vi "Lab Panel V2.1.vi"() -> ()   [LabVIEW 2013]
uses:
  <vilib>/Platform/TimedLoop/XDataNode/timing_clust.ctl
  <vilib>/Platform/TimedLoop/XDataNode/nitl_modes.ctl
  <vilib>/Platform/TimedLoop/XDataNode/wakeup.ctl
  <vilib>/platform/TimedLoop/XDataNode/XDataNode.xnode
  <vilib>/Platform/TimedLoop/XDataNode/XDNodeRunTimeDep.lvlib
panel:
  in  "Tab Control 2":enum32{"Page 1", "Page 2", "ADMIN"}(tab)
  in  "LA05-2 Name":string
  in  "LA05-1 Name":string
  in  "LA01-1 Testers Name 2":string
  in  "LA01-1 Testers Name":string
  in  "LA01-1 Testers Name 6":string
  in  "LA01-1 Testers Name 5":string
  in  "LA01-1 Testers Name 4":string
  in  "LA01-1 Testers Name 3":string
  in  "LA01-2 Name":string
  in  "LA01-1 Name":string
  out "LA01-1 (V) 10":dbl
  out "LA01-1 (V) 9":dbl
  out "LA01-1 (V) 8":dbl
  out "LA01-1 (V) 7":dbl
  out "LA01-1 (V) 6":dbl
  out "LA01-1 (V) 5":dbl
  out "LA01-1 (V) 4":dbl
  out "LA01-1 (V) 3":dbl
  out "LA01-2 (V)":dbl
  out "LA01-1 (V)":dbl
  in  "Tab Control":T1(tab)
  out "Waveform Graph":dynamicdata(graph)
  out "Waveform Graph 2":dynamicdata(graph)
  out "volt1 4":dbl format="%.2g"
  out "volt1 3":dbl format="%.2g"
  out "volt1 2":dbl format="%.2g"
  out "volt1":dbl format="%.2g"
  out "Waveform Graph 3":dynamicdata(graph)
  out "error out":errorcluster
  in  "Stop Button":bool
  out "AI loop time":dbl format="%.6g"
  out "loops":dbl
  out "saving data":bool
  in  "loop  delay(mS)":dbl
  out "Filename Out":path
  out "on loops":dbl
  in  "on time":dbl=1.0 min=1.0 max=10.0 step=0.5 format="%.1g"
  out "off loops":dbl
  in  "off time":dbl=2.0 min=2.0 max=10.0 step=0.5 format="%.1g"
  out "jig":bool
  out "jig cycle":dbl
  in  "run test":bool
  in  "calibrate":bool
  in  "LA01 TEMP":dbl[](array[numeric])
  in  "LA02 TEMP":dbl[](array[numeric])
  in  "LA03 TEMP":dbl[](array[numeric])
  in  "LA04 TEMP":dbl[](array[numeric])
  in  "LA05 TEMP":dbl[](array[numeric])
  in  "TEMP CAL":dbl
  out "AI update":bool
  out "TEMP update":bool
  out "TEMP error":bool
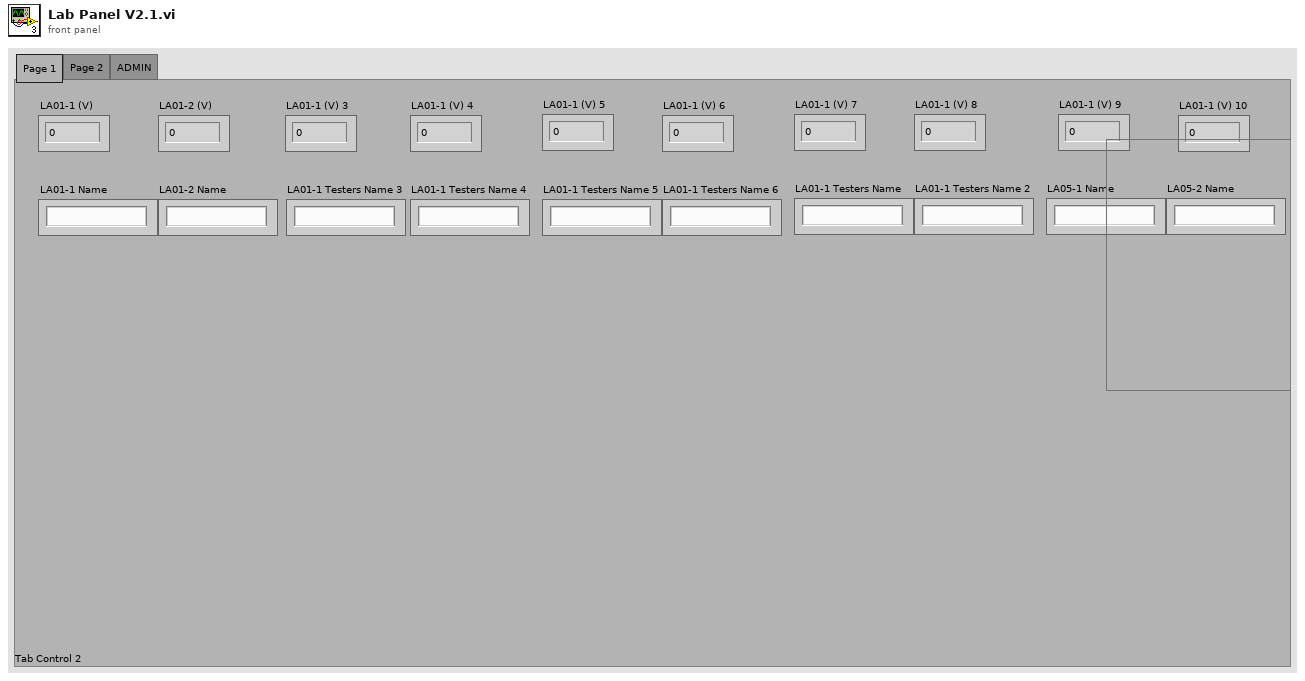
[diagram p1: front panel]
types:
  T1 = enum32{"Page 1", "Page 2", "Page 3", "Page 4", "Page 5"}
  T2 = typedef "XDNodeRunTimeDep.lvlib/timing_clust.ctl" = cluster{"Expected End [f-1]":u64, "Actual End [f-1]":u64, "Finished Late? [f-1]":bool, "Expected End [i-1]":u64, "Actual End [i-1]":u64, "Finished Late? [i-1]":bool, "Expected Start [i]":u64, "Actual Start [i]":u64, "Expected Start [f]":u64, "Actual Start [f]":u64, "Source Name":string, "Structure Name":string, "Period":i64, "Deadline":i64, "Offset":i64, "Start":i64, "Priority":i32, "Timeout":i32, "Mode":T3, "Wakeup Reason":T4, "Error":errorcluster, "Source Type":string, "Secondary Source Type":string, "Global End Time":u64, "Global Start Time":u64, "Frame Duration":u64, "Iteration Duration":u64, "Assigned CPU":i32, "I/O Scan Engine Mode":u32}
  T3 = typedef "XDNodeRunTimeDep.lvlib/nitl_modes.ctl" = enum32{"No Change", "Process missed periods, maintain original phase", "Discard missed periods, maintain original phase", "Process missed periods, ignore original phase", "Discard missed periods, ignore original phase"}
  T4 = typedef "XDNodeRunTimeDep.lvlib/wakeup.ctl" = enum32{"Normal", "Aborted", "Asynchronous wakeup", "Timing source error", "Timed loop error", "Timeout"}
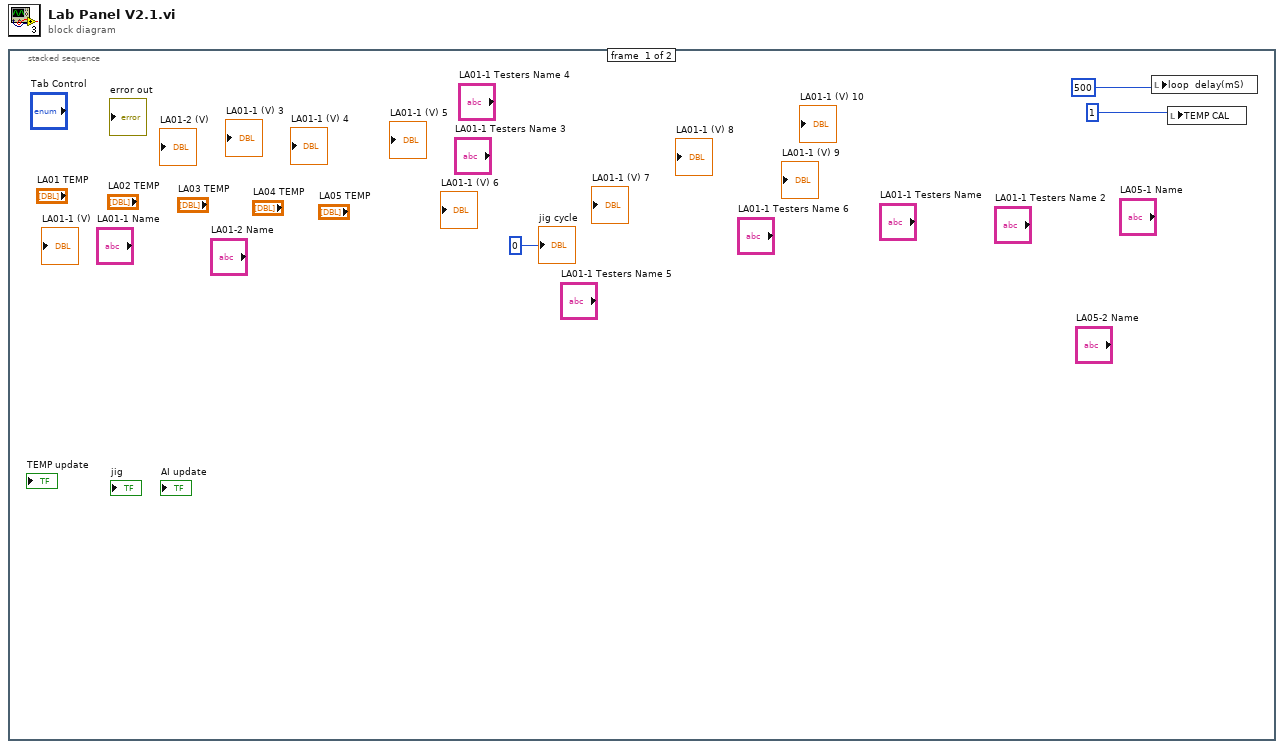
[diagram p0: block diagram]
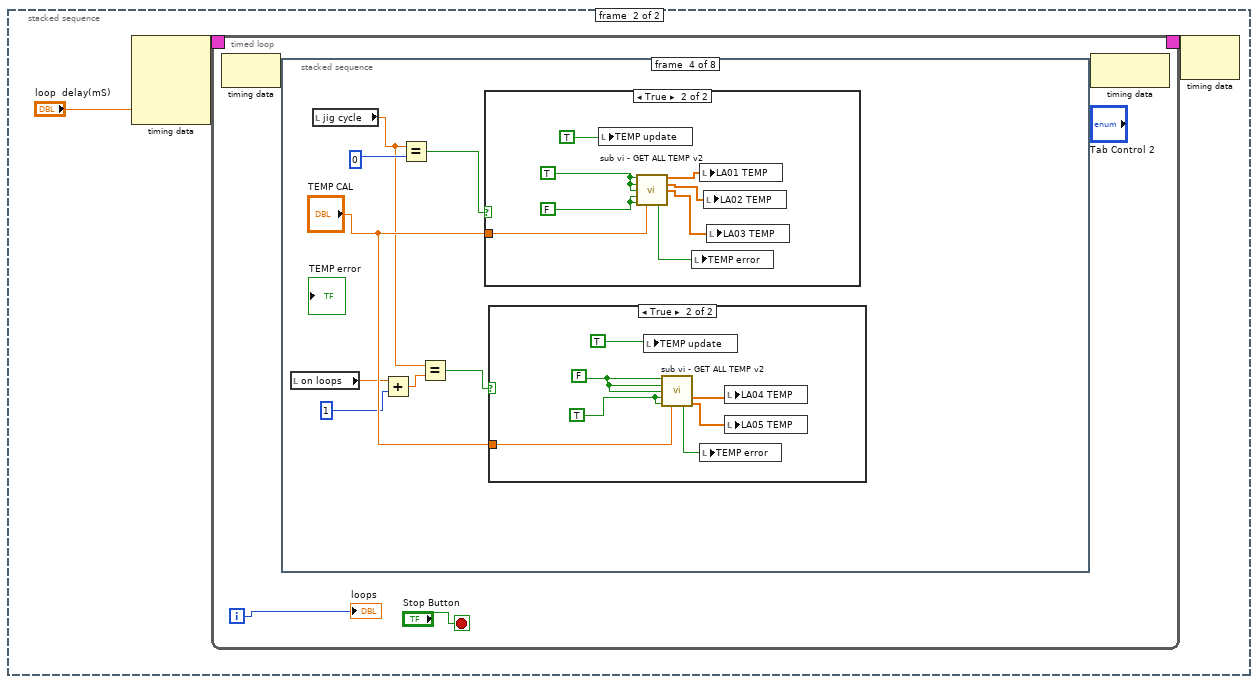
[diagram p2: hidden frame]
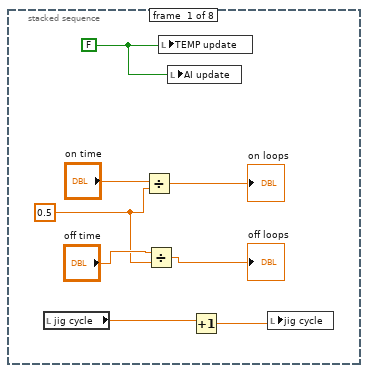
[diagram p3: hidden frame]
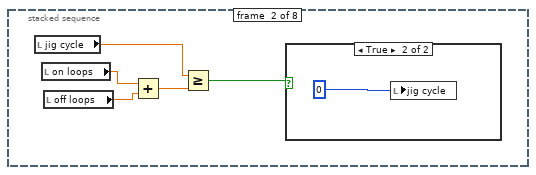
[diagram p4: hidden frame]
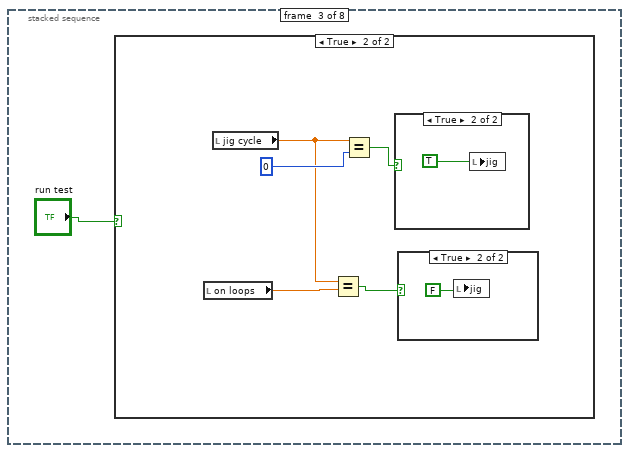
[diagram p6: hidden frame]
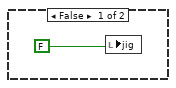
[diagram p7: hidden frame]
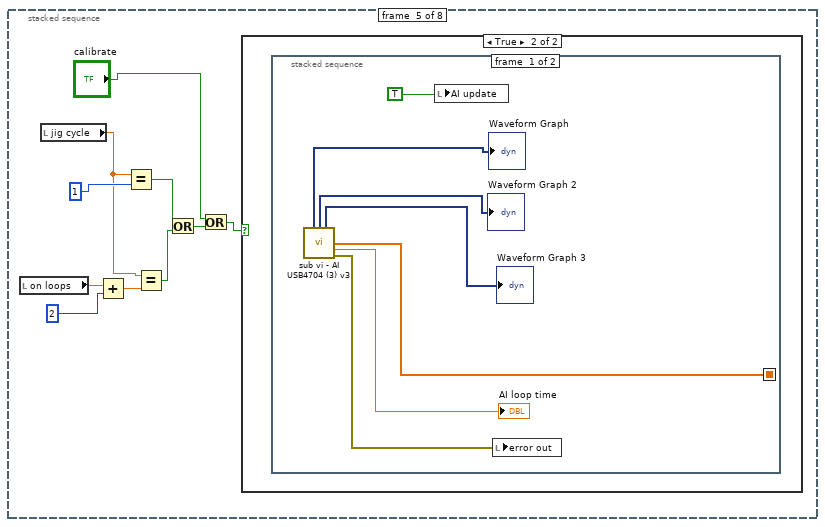
[diagram p12: hidden frame]
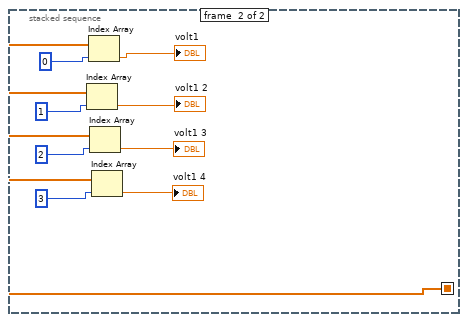
[diagram p14: hidden frame]
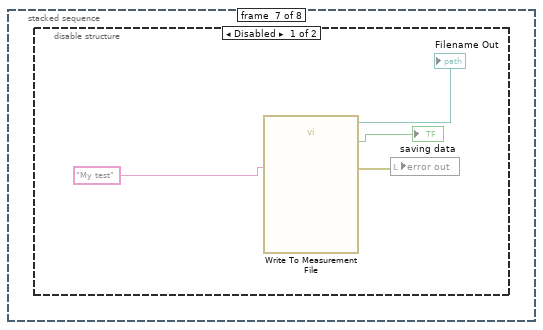
[diagram p16: hidden frame]
diagram:
  n1 = stacked-sequence {
    frame #0 {
      n2 = local write "loop  delay(mS)"(500) -> ()
      n3 = local write "TEMP CAL"(1) -> ()
      "jig cycle" <- 0
    }
    frame #1 {
      n4 = node-c288("loop  delay(mS)") -> (w6:T2)  [unwired: 3 in]
      n5 = timed-loop {
        timing: w6 -> [_]
        timing-out: [_] -> w5
        i -> [w7]
        stop <- "Stop Button" stop-if-true
        n6 = node-c288() -> ()  [unwired: 1 in, 1 out]
        n7 = stacked-sequence {
          frame #0 {
            w11 = FALSE
            w16 = 0.5
            n8 = local read "jig cycle"() -> (w15:dbl)
            n9 = Divide(x="on time", y=w16) -> (x/y=→"on loops":dbl)
            n10 = Divide(x="off time", y=w16) -> (x/y=→"off loops":dbl)
            n11 = local write "TEMP update"(w11) -> ()
            n12 = local write "AI update"(w11) -> ()
            n13 = Increment(x=w15) -> (x+1=w14:dbl)
            n14 = local write "jig cycle"(w14) -> ()
          }
          frame #1 {
            n15 = local read "jig cycle"() -> (w20:dbl)
            n16 = local read "on loops"() -> (w23:dbl)
            n17 = local read "off loops"() -> (w22:dbl)
            n18 = Add(x=w23, y=w22) -> (x+y=w21:dbl)
            n19 = Greater Or Equal?(x=w20, y=w21) -> (x >= y?=w19:bool)
            n20 = case shown="True" w19 {
              frame False {
              }
              frame True {
                n21 = local write "jig cycle"(0) -> ()
              }
            }
          }
          frame #2 {
            n22 = case shown="True" "run test" {
              frame False {
                n23 = local write "jig"(FALSE) -> ()
              }
              frame True {
                n24 = local read "on loops"() -> (w27:dbl)
                n25 = local read "jig cycle"() -> (w29:dbl)
                n26 = Equal?(x=w29, y=w27) -> (x = y?=w28:bool)
                n27 = Equal?(x=w29, y=0) -> (x = y?=w31:bool)
                n28 = case shown="True" w31 {
                  frame False {
                  }
                  frame True {
                    n29 = local write "jig"(TRUE) -> ()
                  }
                }
                n30 = case shown="True" w28 {
                  frame False {
                  }
                  frame True {
                    n31 = local write "jig"(FALSE) -> ()
                  }
                }
              }
            }
          }
          frame #3 {
            n32 = local read "on loops"() -> (w36:dbl)
            n33 = local read "jig cycle"() -> (w38:dbl)
            n34 = Add(x=w36, y=1) -> (x+y=w37:dbl)
            n35 = Equal?(x=w38, y=0) -> (x = y?=w40:bool)
            n36 = Equal?(x=w38, y=w37) -> (x = y?=w34:bool)
            n37 = case shown="True" w40 {
              tunnel: "TEMP CAL" -> [_ w51]
              frame False {
              }
              frame True {
                w55 = FALSE
                w56 = TRUE
                n38 = local write "TEMP update"(TRUE) -> ()
                n39 = call "sub vi - GET ALL TEMP v2.vi"("LA01-EN"=w56, "LA02-EN"=w56, "LA03-EN"=w56, "LA04-EN"=w55, "LA05-EN"=w55, "Gen Cal Value"=w51) -> ("LA01 TEMP"=w54:dbl[], "LA02 TEMP"=w53:dbl[], "LA03 TEMP"=w52:dbl[], "error"=w49:bool)  [unwired: 4 in, 2 out]
                n40 = local write "TEMP error"(w49) -> ()
                n41 = local write "LA01 TEMP"(w54) -> ()
                n42 = local write "LA02 TEMP"(w53) -> ()
                n43 = local write "LA03 TEMP"(w52) -> ()
              }
            }
            n44 = case shown="True" w34 {
              tunnel: "TEMP CAL" -> [_ w48]
              frame False {
              }
              frame True {
                w46 = TRUE
                w47 = FALSE
                n45 = local write "TEMP update"(TRUE) -> ()
                n46 = call "sub vi - GET ALL TEMP v2.vi"("LA01-EN"=w47, "LA02-EN"=w47, "LA03-EN"=w47, "LA04-EN"=w46, "LA05-EN"=w46, "Gen Cal Value"=w48) -> ("LA04 TEMP"=w45:dbl[], "error"=w42:bool, "LA05 TEMP"=w44:dbl[])  [unwired: 4 in, 3 out]
                n47 = local write "TEMP error"(w42) -> ()
                n48 = local write "LA04 TEMP"(w45) -> ()
                n49 = local write "LA05 TEMP"(w44) -> ()
              }
            }
          }
          frame #4 {
            n50 = local read "on loops"() -> (w65:dbl)
            n51 = local read "jig cycle"() -> (w62:dbl)
            n52 = Add(x=w65, y=2) -> (x+y=w63:dbl)
            n53 = Equal?(x=w62, y=1) -> (x = y?=w60:bool)
            n54 = Equal?(x=w62, y=w63) -> (x = y?=w61:bool)
            n55 = Or(x=w60, y=w61) -> (x .or. y?=w59:bool)
            n56 = Or(x="calibrate", y=w59) -> (x .or. y?=w57:bool)
            n57 = case shown="True" w57 {
              frame False {
              }
              frame True {
                n58 = stacked-sequence {
                  seq-local: [w69 _] -> [_ w82]
                  frame #0 {
                    n59 = call "sub vi - AI USB4704 (3) v3.vi"() -> ("Graph 1"=→"Waveform Graph":dynamicdata, "Graph 2"=→"Waveform Graph 2":dynamicdata, "Graph 3"=→"Waveform Graph 3":dynamicdata, "RMS values 3"=w69:dbl[], "loop time"=→"AI loop time":dbl, "error out"=w71:errorcluster)  [unwired: 8 in, 2 out]
                    n60 = local write "AI update"(TRUE) -> ()
                    n61 = local write "error out"(w71) -> ()
                  }
                  frame #1 {
                    n62 = Index Array(array=w82, index=1) -> (element=→"volt1 2":dbl)
                    n63 = Index Array(array=w82, index=0) -> (element=→"volt1":dbl)
                    n64 = Index Array(array=w82, index=2) -> (element=→"volt1 3":dbl)
                    n65 = Index Array(array=w82, index=3) -> (element=→"volt1 4":dbl)
                  }
                }
              }
            }
          }
          frame #5 {
          }
          frame #6 {
            n66 = disable-structure shown="Disabled" {
              frame Disabled {
                n67 = call "Write To Measurement File"("Comment"="My test") -> ("Filename Out"=→"Filename Out":path, "Saving Data"=→"saving data":bool, "error out"=w86:errorcluster)  [unwired: 16 in]
                n68 = local write "error out"(w86) -> ()
              }
              frame Enabled {
              }
            }
          }
          frame #7 {
          }
        }
        n69 = node-c288() -> ()  [unwired: 1 in, 1 out]
        "loops" <- w7
      }
      n70 = node-c288(w5) -> ()  [unwired: 1 out]
    }
  }
